vi "Sort Multi_Run.vi"() -> ()   [LabVIEW 2020]
uses:
  Anemometry Sub Vis/Globals/Extra_Commands_Global.vi
  Anemometry Sub Vis/Globals/Trav_pos_global.vi
  Anemometry Sub Vis/Controls/Tunnel_Coordinates.ctl
panel:
  out "Work in Tunnel Coordinates?":T1
  in  "Command filename":path
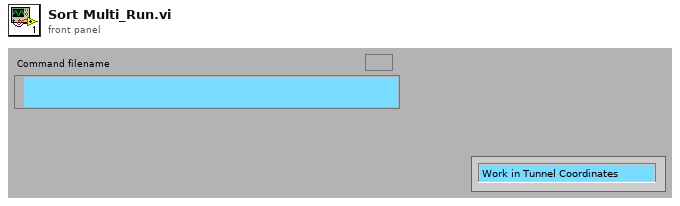
[diagram p1: front panel]
types:
  T1 = typedef "Tunnel_Coordinates.ctl" = enum16{"Work in Tunnel Coordinates", "Work in Model Coordinates"}
  T2 = typedef "Traverse_cluster.ctl" = cluster{"Start X":sgl, "Start Y":sgl, "Start Z":sgl, "End X":sgl, "End Y":sgl, "End Z":sgl, "No. of pts.":i32, "Spacing":T3, "Filename":path, "Tunnel Speed":dbl, "Averaging time (mins)":dbl, "Extra Commands":string, "Carrier_1 Q (l/min)":dbl, "Carrier_2 Q (l/min)":dbl, "Trace Gas Concentration (%)":dbl, "Specific Arguments":string, "Comments":string, "Row No":i32, "Row Type Selector":T4, "EstCompl":string, "Row Duration (mins)":dbl, "No. of Valid pts.":i32, "Meas Setup File":string}
  T3 = typedef "Spacing.ctl" = enum16{"Linear", "Log", "Gauss", "Specified", "N/A"}
  T4 = typedef "Multi_run_mode.ctl" = enum16{"Move Traverse Only", "Set Tunnel Speed Only", "Set Source Only", "Set Measurement Conditions", "Single Measurement", "Vertical Profile", "Lateral Profile", "Longitudinal Profile", "Multi-Axis Profile", "Explore Volume", "Auto Calibrate", "Meas Fast FID Bkgnd", "Check Beam Power", "Scanning Valve Measurement", "Run VI Named:", "Set ADAM Ch", "Wait (minutes)", "Send Message", "Synchronize With:", "Fall Back to this Row", "Turn Off Row Repeating", "Traverse 3D Volume", "Blank Row", "Jump to Fall Back Row"}
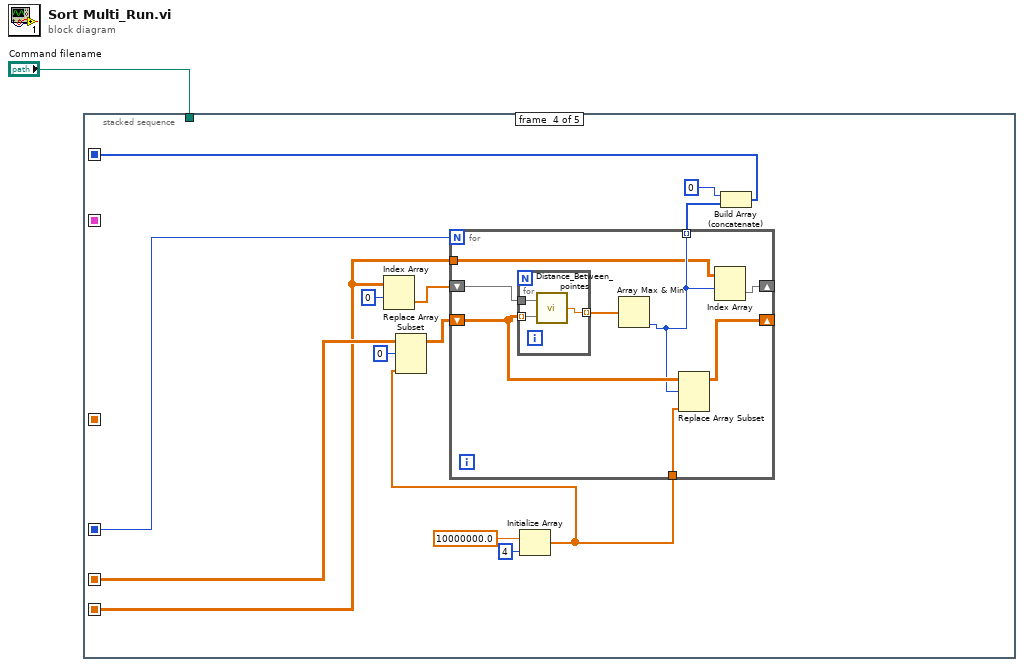
[diagram p0: block diagram]
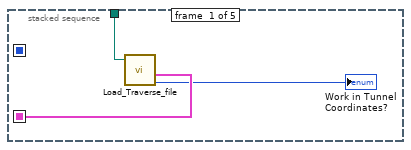
[diagram p2: hidden frame]
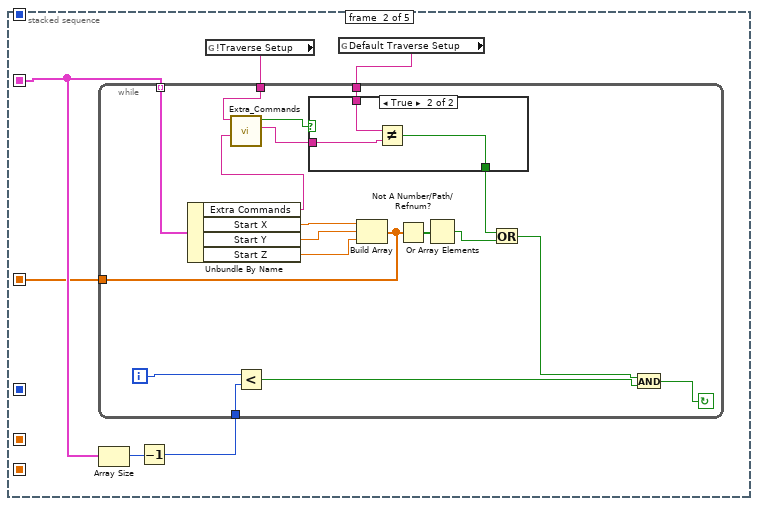
[diagram p3: hidden frame]
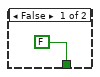
[diagram p4: hidden frame]
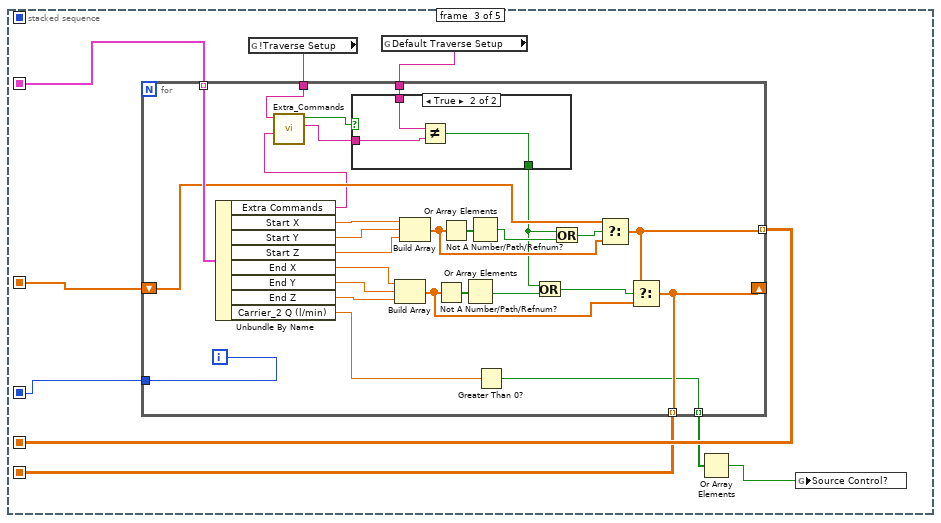
[diagram p5: hidden frame]
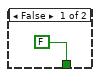
[diagram p6: hidden frame]
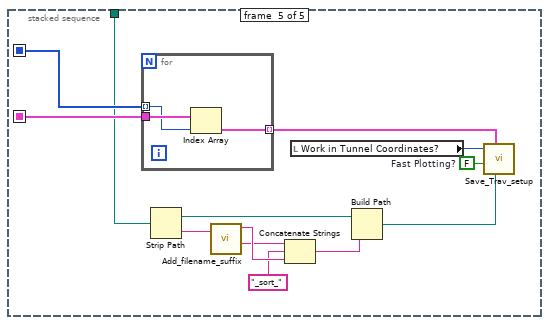
[diagram p7: hidden frame]
diagram:
  n1 = stacked-sequence {
    seq-local: [_ _ w41 _ _] -> [_ _ _ w79 _]
    seq-local: [_ _ w40 _ _] -> [_ _ _ w78 _]
    seq-local: [_ _ w39 _ _] -> [_ _ _ w77 _]
    seq-local: [_ _ _ w74 _] -> [_ _ _ _ w108]
    seq-local: [w3 _ _ _ _] -> [_ w8 w38 _ w109]
    seq-local: [_ w5 _ _ _] -> [_ _ w35 _ _]
    tunnel: "Command filename" -> [w4 _ _ _ w106]
    frame #0 {
      n2 = call "Load_Traverse_file.vi"("Setup filename"=w4) -> ("Table"=w3:T2[], "Work in Tunnel Coordinates?"=→"Work in Tunnel Coordinates?":T1)  [unwired: 4 out]
    }
    frame #1 {
      n3 = Array Size(array=w8) -> (size(s)=w7:i32)
      n4 = Decrement(x=w7) -> (x-1=w6:i32)
      n5 = global read "Extra_Commands_Global.vi" "!Traverse Setup"() -> (w10:string)
      n6 = global read "Trav_pos_global.vi" "Default Traverse Setup"() -> (w9:string)
      n7 = while {
        tunnel: w8 -> [w28] mode=indexing
        tunnel: w10 -> [w23]
        tunnel: w9 -> [w19]
        tunnel: w6 -> [w15]
        tunnel: [w12] -> w5
        i -> [w16]
        stop <- w11 continue-if-true
        n8 = Unbundle By Name(w28) -> ("Extra Commands"=w22:string, "Start X"=w26:sgl, "Start Y"=w25:sgl, "Start Z"=w24:sgl)
        n9 = call "Extra_Commands.vi"("String to Search"=w22, "Command"=w23) -> ("String Value"=w20:string, "Command Found"=w21:bool)  [unwired: 1 in, 3 out]
        n10 = Less?(x=w16, y=w15) -> (x < y?=w14:bool)
        n11 = case shown="True" w21 {
          tunnel: w20 -> [_ w32]
          tunnel: w19 -> [_ w31]
          tunnel: [FALSE w30] -> w17
          frame False {
          }
          frame True {
            n12 = Not Equal?(x=w31, y=w32) -> (x != y?=w30:bool)
          }
        }
        n13 = Build Array(w26, w25, w24) -> (w12:sgl[])
        n14 = Not A Number/Path/Refnum?(number/path/refnum=w12) -> (NaN/Path/Refnum?=w27:bool[])
        n15 = Or Array Elements(Boolean array=w27) -> (logical OR=w18:bool)
        n16 = Or(x=w17, y=w18) -> (x .or. y?=w13:bool)
        n17 = And(x=w13, y=w14) -> (x .and. y?=w11:bool)
      }
    }
    frame #2 {
      n18 = global read "Extra_Commands_Global.vi" "!Traverse Setup"() -> (w37:string)
      n19 = global read "Trav_pos_global.vi" "Default Traverse Setup"() -> (w36:string)
      n20 = for {
        tunnel: w38 -> [w68] mode=indexing
        shift-right: [w55] -> _
        shift-left: w35 -> [w56]
        tunnel: [w57] -> w41 mode=indexing
        tunnel: [w55] -> w40 mode=indexing
        tunnel: [w54] -> w39
        tunnel: w37 -> [w53]
        tunnel: w36 -> [w49]
        tunnel: [w42] -> w33 mode=indexing
        i -> [w54]
        n21 = Unbundle By Name(w68) -> ("Extra Commands"=w52:string, "Start X"=w66:sgl, "Start Y"=w65:sgl, "Start Z"=w64:sgl, "End X"=w60:sgl, "End Y"=w59:sgl, "End Z"=w58:sgl, "Carrier_2 Q (l/min)"=w43:dbl)
        n22 = call "Extra_Commands.vi"("String to Search"=w52, "Command"=w53) -> ("String Value"=w50:string, "Command Found"=w51:bool)  [unwired: 1 in, 3 out]
        n23 = case shown="True" w51 {
          tunnel: w50 -> [_ w72]
          tunnel: w49 -> [_ w71]
          tunnel: [FALSE w70] -> w45
          frame False {
          }
          frame True {
            n24 = Not Equal?(x=w71, y=w72) -> (x != y?=w70:bool)
          }
        }
        n25 = Build Array(w60, w59, w58) -> (w62:sgl[])
        n26 = Build Array(w66, w65, w64) -> (w63:sgl[])
        n27 = Not A Number/Path/Refnum?(number/path/refnum=w62) -> (NaN/Path/Refnum?=w61:bool[])
        n28 = Not A Number/Path/Refnum?(number/path/refnum=w63) -> (NaN/Path/Refnum?=w67:bool[])
        n29 = Or Array Elements(Boolean array=w61) -> (logical OR=w46:bool)
        n30 = Or Array Elements(Boolean array=w67) -> (logical OR=w47:bool)
        n31 = Greater Than 0?(x=w43) -> (x > 0?=w42:bool)
        n32 = Or(x=w45, y=w46) -> (x .or. y?=w44:bool)
        n33 = Or(x=w45, y=w47) -> (x .or. y?=w48:bool)
        n34 = Select(t=w56, s=w48, f=w63) -> (s? t:f=w57:sgl[])
        n35 = Select(t=w57, s=w44, f=w62) -> (s? t:f=w55:sgl[])
      }
      n36 = Or Array Elements(Boolean array=w33) -> (logical OR=w34:bool)
      n37 = global write "Trav_pos_global.vi" "Source Control?"(w34) -> ()
    }
    frame #3 {
      n38 = Index Array(array=w78, index (row)=0) -> (element=w81:sgl[])  [unwired: 1 in]
      n39 = Initialize Array(10000000.0 ("element"), 4 ("dimension size")) -> (w84:dbl[])
      n40 = Replace Array Subset(array=w79, new element=w84, index (row)=0) -> (w85:sgl[][])  [unwired: 1 in]
      n41 = for {
        N: w77 -> [_]
        tunnel: [w88] -> w75 mode=indexing
        shift-right: [w91] -> _
        shift-left: w85 -> [w92]
        shift-right: [w89] -> _
        shift-left: w81 -> [w90]
        tunnel: w78 -> [w87]
        tunnel: w84 -> [w86]
        n42 = for {
          tunnel: w90 -> [w96]
          tunnel: w92 -> [w95] mode=indexing
          tunnel: [w94] -> w93 mode=indexing
          n43 = call "Distance_Between_pointes.vi"("P2"=w95, "P1"=w96) -> ("Distance"=w94:dbl)
        }
        n44 = Array Max & Min(array=w93) -> (min index (indices)=w88:i32)  [unwired: 3 out]
        n45 = Replace Array Subset(array=w92, new element=w86, index (row)=w88) -> (w91:sgl[][])  [unwired: 1 in]
        n46 = Index Array(array=w87, index (row)=w88) -> (element=w89:sgl[])  [unwired: 1 in]
      }
      n47 = Build Array (concatenate)(0 ("min index(es)"), w75) -> (w74:i32[])
    }
    frame #4 {
      w97 = FALSE  # Fast Plotting?
      n48 = for {
        tunnel: w109 -> [w112]
        tunnel: w108 -> [w111] mode=indexing
        tunnel: [w110] -> w107 mode=indexing
        n49 = Index Array(array=w112, index=w111) -> (element=w110:T2)
      }
      n50 = Strip Path(path=w106) -> (stripped path=w105:path, name=w104:string)
      n51 = call "Add_filename_suffix.vi"("Filename"=w104) -> ("Original Suffix"=w103:string, "Base name"=w98:string)  [unwired: 1 in, 2 out]
      n52 = Concatenate Strings(w98, "_sort_" ("string"), w103) -> (w101:string)
      n53 = local read "Work in Tunnel Coordinates?"() -> (w99:T1)
      n54 = Build Path(base path=w105, name or relative path=w101) -> (appended path=w100:path)
      n55 = call "Save_Trav_setup.vi"("Work in Tunnel Coordinates?"=w99, "Trav Table"=w107, "Fast Plotting?"=w97, "Setup filename"=w100) -> ()  [unwired: 1 in, 1 out]
    }
  }
